vi "Update Bookmarks View.vi"(8 "Error In":errorcluster, 11 "State In":T1) -> (0 "Error Out":errorcluster, 3 "State Out":T1)   [LabVIEW 2018, in "Bookmark Manager.lvlib"]
uses:
  Bookmark Manager.lvlib
  Controls/State.ctl
  <vilib>/addons/analyzer/_analyzerctrls.llb/VIAnCtl Analysis App Info.ctl
  Controls/Bookmark.ctl
  Controls/VI Identifier.ctl
  Controls/Bookmarks Groups.ctl
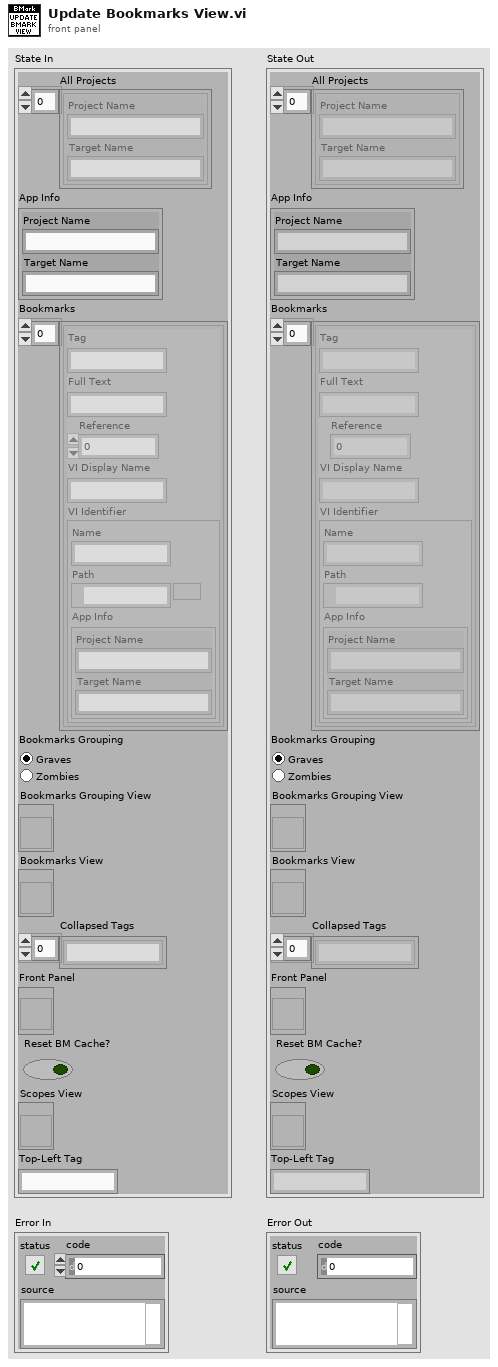
[diagram p1: front panel]
types:
  T1 = typedef "Bookmark Manager.lvlib/State.ctl" = cluster{"All Projects":T2[], "App Info":T2, "Bookmarks":T3[], "Bookmarks Grouping":T5, "Bookmarks Grouping View":refnum<vi>, "Bookmarks View":refnum<vi>, "Collapsed Tags":string[], "Front Panel":refnum<vi>, "Reset BM Cache?":bool, "Scopes View":refnum<vi>, "Top-Left Tag":string}
  T2 = typedef "VIAnCtl Analysis App Info.ctl" = cluster{"Project Name":string, "Target Name":string}
  T3 = typedef "Bookmark Manager.lvlib/Bookmark.ctl" = cluster{"Tag":string, "Full Text":string, "Reference":i32, "VI Display Name":string, "VI Identifier":T4}
  T4 = typedef "Bookmark Manager.lvlib/VI Identifier.ctl" = cluster{"Name":string, "Path":path, "App Info":T2}
  T5 = typedef "Bookmark Manager.lvlib/Bookmarks Groups.ctl" = enum32{"Graves", "Zombies"}
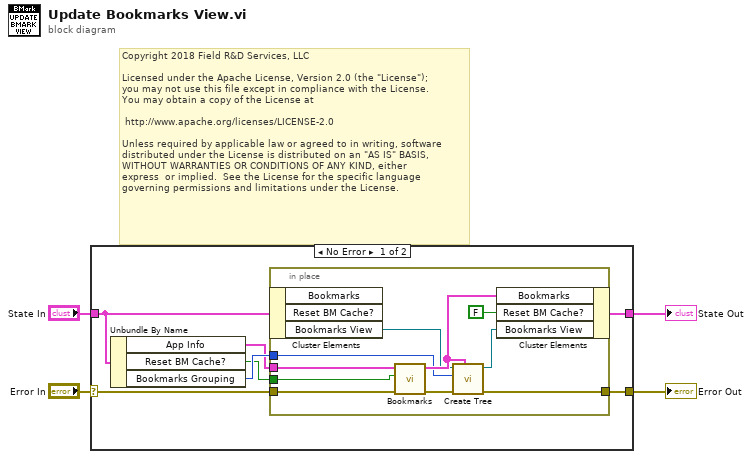
[diagram p0: block diagram]
diagram:
  # "Copyright 2018 Field R&D Services, LLC\n\nLicensed under the Apache License, Version 2.0 (the \"License\");\nyou may not use this file except in compliance with the License.\nYou may obtain a copy of the License at\n\n\thttp://www.apache.org/licenses/LICENSE-2.0\n\nUnless required by applicable law or agreed to in writing, software\ndistributed under the License is distributed on an \"AS IS\" BASIS,\nWITHOUT WARRANTIES OR CONDITIONS OF ANY KIND, either \nexpress  or implied.  See the License for the specific language \ngoverning permissions and limitations under the License."
  n1 = case shown="No Error" "Error In" {
    selector: "Error In" -> [w5 w22]
    tunnel: [w11 w22] -> w4
    tunnel: "State In" -> [w7 w23]
    tunnel: [w6 w23] -> w2
    frame No Error {
      n2 = Unbundle By Name(w7) -> ("App Info"=w8:T2, "Reset BM Cache?"=w9:bool, "Bookmarks Grouping"=w10:T5)
      n3 = in-place {
        in-place-border: w8 -> [w20]
        in-place-border: w9 -> [w19]
        in-place-border: w10 -> [w12]
        in-place-border: w5 -> [w18]
        in-place-border: [w15] -> w11
        n4 = in-place-cluster #1(w7) -> ("Bookmarks View"=w14:refnum<vi>)  [unwired: 2 out]
        n5 = call "Bookmarks.vi"("Error In"=w18, "Reset BM Cache?"=w19, "App Info"=w20) -> ("Error Out"=w16:errorcluster, "Bookmarks"=w17:T3[])  [unwired: 6 in, 1 out]
        n6 = call "Create Tree.vi"("Bookmarks"=w17, "Error In"=w16, "Bookmarks Grouping"=w12, "Bookmarks View In"=w14) -> ("Error Out"=w15:errorcluster, "Bookmarks View Out"=w13:refnum<vi>)  [unwired: 6 in]
        n7 = in-place-cluster #1("Bookmarks"=w17, "Reset BM Cache?"=FALSE, "Bookmarks View"=w13) -> (w6:T1)
      }
    }
    frame Error {
    }
  }
  "Error Out" <- w4
  "State Out" <- w2
